vi "Telescope Simulator Config GUI.vi"(11 "Time to Move Between Positions":dbl) -> (2 "Cancelled":bool, 3 "Time out":dbl)   [LabVIEW 2021, in "Telescope Simulator.lvclass"]
uses:
  Telescope Simulator.lvclass
panel:
  in  "Cancel Button":bool
  in  "OK Button":bool
  # "Seconds"
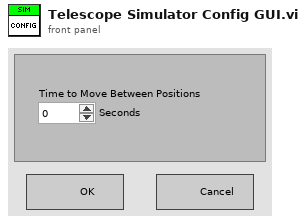
[diagram p1: front panel]
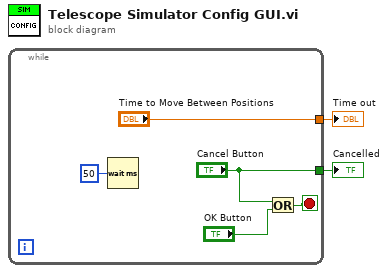
[diagram p0: block diagram]
diagram:
  n1 = while {
    tunnel: ["Cancel Button"] -> w2
    tunnel: ["Time to Move Between Positions"] -> w1
    stop <- w6 stop-if-true
    n2 = Wait (ms)(milliseconds to wait=u32 50) -> ()  [unwired: 1 out]
    n3 = Or(x="Cancel Button", y="OK Button") -> (x .or. y?=w6:bool)
  }
  "Cancelled" <- w2
  "Time out" <- w1
